vi "ReadAmplifierInputOffset.vi"(8 "error in (no error)":errorcluster, 11 "AmplifierSim in":refnum<class "AmplifierSim.lvclass">) -> (0 "error out":errorcluster, 2 "Input Offset":dbl, 3 "AmplifierSim out":refnum<class "AmplifierSim.lvclass">)   [LabVIEW 2017, in "AmplifierSim.lvclass"]
uses:
  AmplifierSim.lvclass
  AmplifierSim.lvclass/AmplifierSim.ctl
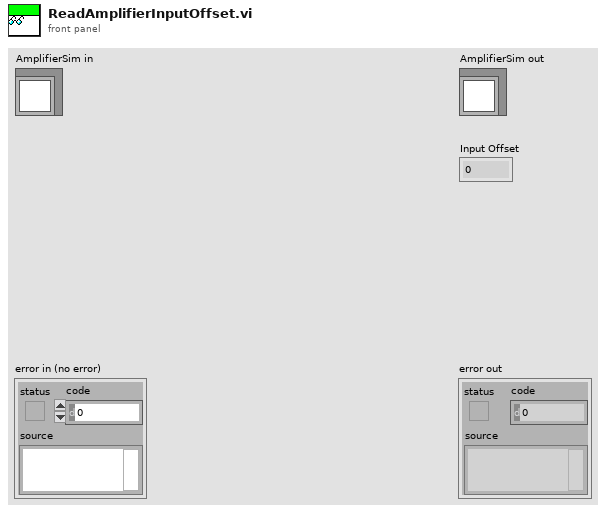
[diagram p1: front panel]
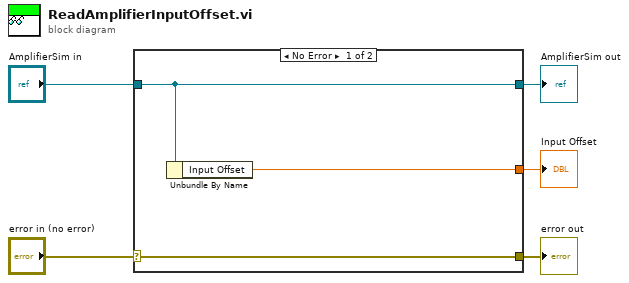
[diagram p0: block diagram]
diagram:
  n1 = case shown="No Error" "error in (no error)" {
    selector: "error in (no error)" -> [w8 w9]
    tunnel: [w8 w9] -> w4
    tunnel: [w7 w10] -> w2
    tunnel: "AmplifierSim in" -> [w7 w10]
    tunnel: [w6 _] -> w1
    frame No Error {
      n2 = Unbundle By Name(w7) -> ("Input Offset"=w6:dbl)
    }
    frame Error {
    }
  }
  "error out" <- w4
  "AmplifierSim out" <- w2
  "Input Offset" <- w1
